vi "CreatePriorityQueue.vi"(8 "error in (no error)":errorcluster) -> (0 "error out":errorcluster, 3 "PriorityQueue":refnum<data-value>)   [LabVIEW 2014, in "PriorityQueue.lvclass"]
uses:
  <userlib>/AdvancedDataStructures/ClassBased/Applications/PriorityQueue/PriorityQueue/PriorityQueue.lvclass
  <userlib>/AdvancedDataStructures/ClassBased/Common/BasicSortedList/BasicSortedList/BasicSortOptions.ctl
  <userlib>/AdvancedDataStructures/ClassBased/Applications/PriorityQueue/PriorityQueue/PriorityQueue.lvclass/PriorityQueue.ctl
  <userlib>/AdvancedDataStructures/ClassBased/Common/BasicSortedList/BasicSortedList/BasicSortedList.lvclass
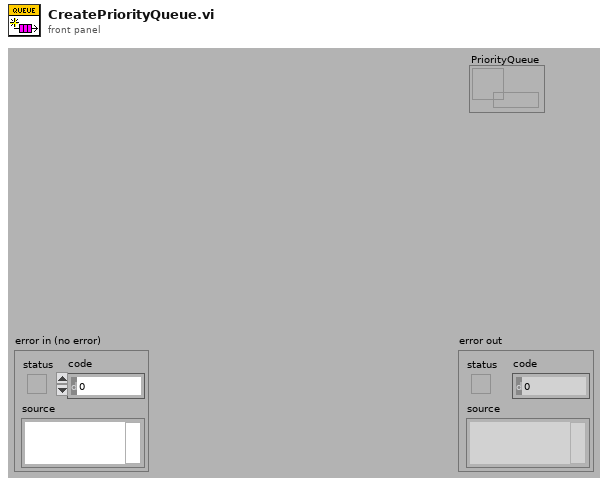
[diagram p1: front panel]
types:
  T1 = typedef "BasicSortedList.lvclass/BasicSortOptions.ctl" = enum16{"Ascending", "Decending"}
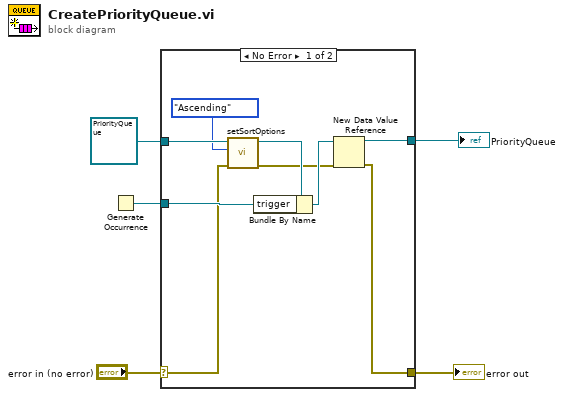
[diagram p0: block diagram]
diagram:
  n1 = Generate Occurrence() -> (w1:refnum<k4>)
  n2 = case shown="No Error" "error in (no error)" {
    selector: "error in (no error)" -> [w7 w15]
    tunnel: [w14 w15] -> w4
    tunnel: [w13 _] -> w3
    tunnel: refnum<class "PriorityQueue.lvclass"> refnum ("PriorityQueue.lvclass") -> [w10 _]
    tunnel: w1 -> [w12 _]
    frame No Error {
      n3 = call <userlib>:"setSortOptions.vi"("error in (no error)"=w7, "SortOptions"=BasicSortOptions."Ascending", "BasicSortedList in"=w10) -> ("error out"=w8:errorcluster, "BasicSortedList out"=w9:refnum<class "PriorityQueue.lvclass">)  [unwired: 7 in]
      n4 = Bundle By Name(cluster=w9, "trigger"=w12) -> (w11:refnum<class "PriorityQueue.lvclass">)
      n5 = New Data Value Reference(data value=w11, error in=w8) -> (data value reference=w13:refnum<data-value>, error out=w14:errorcluster)
    }
    frame Error {
    }
  }
  "error out" <- w4
  "PriorityQueue" <- w3
